vi "PQfnumber.vi"(6 "error in (no error)":errorcluster, 7 "field_name":string, 9 "res":u32) -> (0 "error out":errorcluster, 2 "column_number":u32, 3 "res_out":u32)   [LabVIEW 2019, in "libpqlv.lvlib"]
doc: "Returns the column number associated with the given column name."
uses:
  libpqlv.lvlib
  libpq.dll
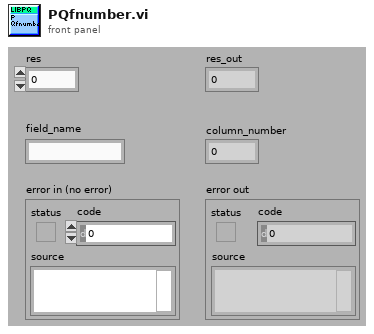
[diagram p1: front panel]
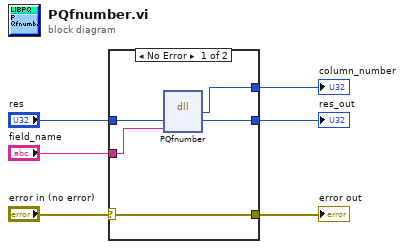
[diagram p0: block diagram]
diagram:
  n1 = case shown="No Error" "error in (no error)" {
    selector: "error in (no error)" -> [w11 w13]
    tunnel: [w11 w13] -> w5
    tunnel: [w10 _] -> w4
    tunnel: "field_name" -> [w9 _]
    tunnel: "res" -> [w8 w12]
    tunnel: [w7 w12] -> w1
    frame No Error {
      n2 = dll-call lib="libpq.*" fn="PQfnumber"("res"=w8, "field_name"=w9) -> ("fnumber"=w10:u32, "res"=w7:u32)  [unwired: 4 in, 2 out]
    }
    frame Error {
    }
  }
  "column_number" <- w4
  "error out" <- w5
  "res_out" <- w1
